vi "startIVAndWait.vi"(8 "error in (no error)":errorcluster, 11 "Instrument.Lockin in":refnum<class "Instrument.Lockin.lvclass">) -> (0 "error out":errorcluster, 2 "AI Waveform":waveform(dbl)[](array[waveform]), 3 "Instrument.Lockin out":refnum<class "Instrument.Lockin.lvclass">)   [LabVIEW 2016, in "Instrument.Lockin.lvclass"]
uses:
  Instrument.Lockin.lvclass
  <vilib>/Utility/error.llb/Error Cluster From Error Code.vi
  <vilib>/ErrorRing/Error Ring.xnode
panel:
  in  "stop":bool
  out "timer (s)":dbl=1.2239999771118164
  # "This VI triggers the lockin and waits until the acquisition is complete"
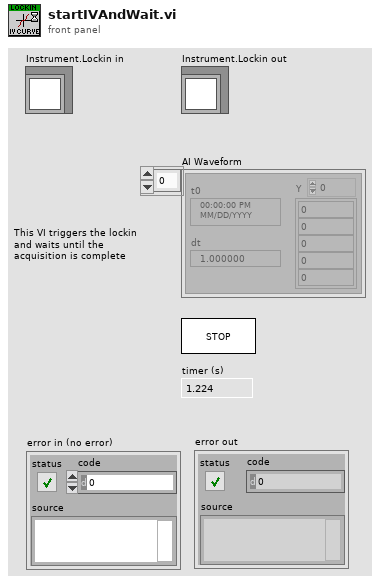
[diagram p1: front panel]
types:
  T1 = typedef "LockinDAQ.lvclass/AO-cluster.ctl" = cluster{"Ch":i32[], "Amp (V)":dbl[], "DC (V)":dbl[], "f (Hz)":dbl[], "Phase (°)":dbl[], "Function":T2[], "Sweep?":bool[]}
  T2 = typedef "LockinDAQ.lvclass/Function-enum.ctl" = enum16{"Sine", "Triangle", "Square", "Sawtooth"}
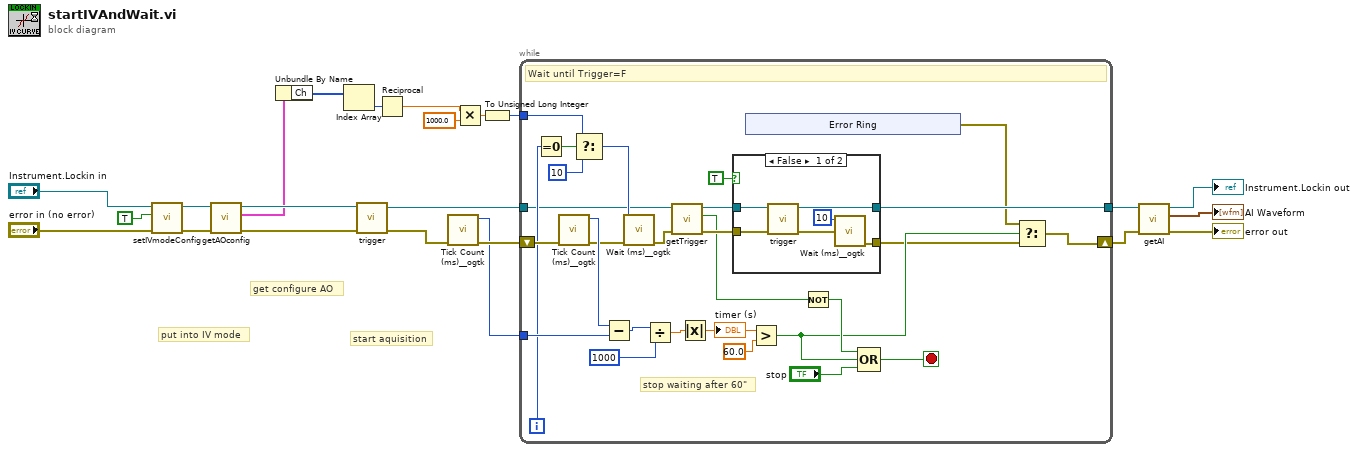
[diagram p0: block diagram]
diagram:
  # "start aquisition"
  # "get configure AO"
  # "put into IV mode"
  n1 = call "setIVmodeConfig.vi"("error in (no error)"="error in (no error)", "IV mode"=TRUE, "Instrument.Lockin in"="Instrument.Lockin in") -> ("error out"=w8:errorcluster, "Instrument.Lockin out"=w7:refnum<class "Instrument.Lockin.lvclass">)  [unwired: 7 in]
  n2 = call "getAOconfig.vi"("error in (no error)"=w8, "Instrument.Lockin in"=w7) -> ("error out"=w6:errorcluster, "AOconfig"=w3:T1, "Instrument.Lockin out"=w5:refnum<class "Instrument.Lockin.lvclass">)  [unwired: 7 in]
  n3 = Unbundle By Name(w3) -> ("Ch"=w19:i32[])
  n4 = Index Array(array=w19) -> (element=w18:i32)  [unwired: 1 in]
  n5 = call "trigger.vi"("error in (no error)"=w6, "Instrument.Lockin in"=w5) -> ("error out"=w4:errorcluster, "Instrument.Lockin out"=w10:refnum<class "Instrument.Lockin.lvclass">)  [unwired: 8 in]
  n6 = Reciprocal(x=w18) -> (1/x=w15:dbl)
  n7 = call <userlib>:"Tick Count (ms)__ogtk.vi"("error in (no error)"=w4) -> ("error out"=w22:errorcluster, "millisecond timer value"=w21:u32)  [unwired: 9 in]
  n8 = Multiply(x=w15, y=1000.0) -> (x*y=w16:dbl)
  n9 = To Unsigned Long Integer(number=w16) -> (unsigned 32bit integer=w14:u32)
  n10 = while {
    shift-right: [w28] -> w2
    shift-left: w22 -> [w49]
    tunnel: w21 -> [w47]
    tunnel: w14 -> [w35]
    tunnel: [w33] -> w11
    tunnel: w10 -> [w31]
    i -> [w39]
    stop <- w45 stop-if-true
    # "stop waiting after 60\""
    # "Wait until Trigger=F"
    n11 = Equal To 0?(x=w39) -> (x = 0?=w38:bool)
    n12 = call <userlib>:"Tick Count (ms)__ogtk.vi"("error in (no error)"=w49) -> ("error out"=w42:errorcluster, "millisecond timer value"=w48:u32)  [unwired: 9 in]
    n13 = Select(t=w35, s=w38, f=u32 10) -> (s? t:f=w36:u32)
    n14 = Subtract(x=w48, y=w47) -> (x-y=w24:u32)
    n15 = call <userlib>:"Wait (ms)__ogtk.vi"("error in (no error)"=w42, "milliseconds to wait"=w36) -> ("error out"=w41:errorcluster)  [unwired: 8 in, 1 out]
    n16 = Divide(x=w24, y=u32 1000 ("x")) -> (x/y=w26:dbl)
    n17 = call "getTrigger.vi"("error in (no error)"=w41, "Instrument.Lockin"=w31) -> ("error out"=w44:errorcluster, "Trigger"=w34:bool, "Instrument.Lockin"=w32:refnum<class "Instrument.Lockin.lvclass">)  [unwired: 7 in]
    n18 = Absolute Value(x=w26) -> (abs(x)=w50:dbl)
    "timer (s)" <- w50
    n19 = case shown="False" TRUE {
      tunnel: w44 -> [w61 w63]
      tunnel: [w58 w63] -> w29
      tunnel: [w57 w62] -> w33
      tunnel: w32 -> [w56 w62]
      frame False {
        n20 = call "trigger.vi"("error in (no error)"=w61, "Instrument.Lockin in"=w56) -> ("error out"=w59:errorcluster, "Instrument.Lockin out"=w57:refnum<class "Instrument.Lockin.lvclass">)  [unwired: 8 in]
        n21 = call <userlib>:"Wait (ms)__ogtk.vi"("error in (no error)"=w59, "milliseconds to wait"=u32 10) -> ("error out"=w58:errorcluster)  [unwired: 8 in, 1 out]
      }
      frame True {
      }
    }
    n22 = xnode "Error Ring"() -> ("error out"=w27:errorcluster)
    n23 = Greater?(x=w50, y=60.0) -> (0:w30:bool)
    n24 = Not(x=w34) -> (.not. x?=w46:bool)
    n25 = Compound Arithmetic op=OR(w46, w30, "stop") -> (w45:bool)
    n26 = Select(t=w27, s=w30, f=w29) -> (s? t:f=w28:errorcluster)
  }
  n27 = call "getAI.vi"("error in (no error)"=w2, "Instrument.Lockin in"=w11) -> ("error out"=→"error out":errorcluster, "AI Waveform"=→"AI Waveform":waveform(dbl)[], "Instrument.Lockin out"=→"Instrument.Lockin out":refnum<class "Instrument.Lockin.lvclass">)  [unwired: 7 in]
